vi "ArrayofStrings_to_MultilineString.vi"(0 "String Array":string[](array[string]), 1 "NewLineString":string="\n") -> (2 "String 1":string)   [LabVIEW 2011]
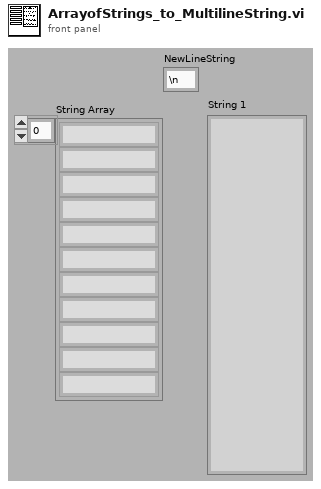
[diagram p1: front panel]
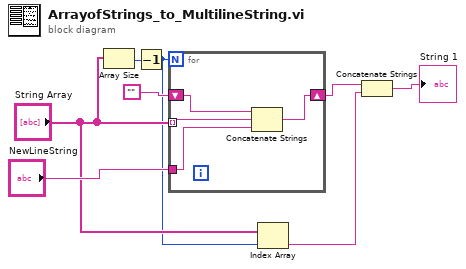
[diagram p0: block diagram]
diagram:
  n1 = Array Size(array="String Array") -> (size(s)=w5:i32)
  n2 = Decrement(x=w5) -> (x-1=w1:i32)
  n3 = for {
    N: w1 -> [_]
    tunnel: "String Array" -> [w11] mode=indexing
    shift-right: [w9] -> w6
    shift-left: "" -> [w12]
    tunnel: "NewLineString" -> [w10]
    n4 = Concatenate Strings(w12, w11, w10) -> (w9:string)
  }
  n5 = Index Array(array="String Array", index=w1) -> (element=w2:string)
  n6 = Concatenate Strings(w6, w2) -> (→"String 1":string)
